vi "FMA1600A Get Total Flow.vi"(6 "Timer":dbl, 8 "error in (no error)":errorcluster, 9 "Min to Sec Convert (Total Flow)":dbl=60.0, 10 "LPM (Vol. Flow)":dbl, 11 "Integral Array Input":dbl[](array[numeric])) -> (0 "error out":errorcluster, 2 "Integral":dbl, 3 "Integral Array Output":dbl[](array[numeric]))   [LabVIEW 2016]
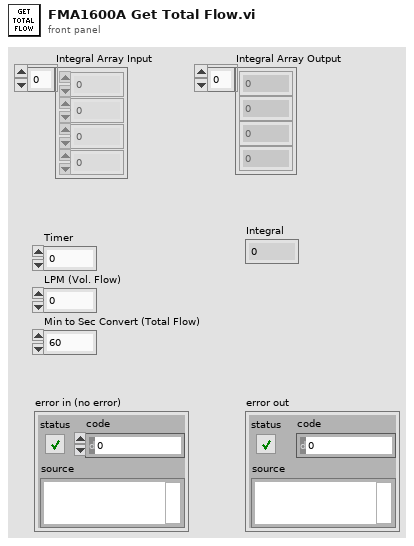
[diagram p1: front panel]
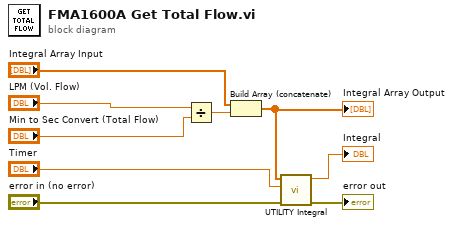
[diagram p0: block diagram]
diagram:
  n1 = Divide(x="LPM (Vol. Flow)", y="Min to Sec Convert (Total Flow)") -> (x/y=w8:dbl)
  n2 = Build Array (concatenate)("Integral Array Input", w8) -> (w2:dbl[])
  "Integral Array Output" <- w2
  n3 = call "UTILITY Integral.vi"("Error In"="error in (no error)", "dt"="Timer", "Array Input"=w2) -> ("Error Out"=→"error out":errorcluster, "Integral"=→"Integral":dbl)  [unwired: 7 in]
